vi "Meas Loop.vi"(8 "error in":errorcluster, 11 "meas in":T1={"swp cfg"={"N"=0, "R"=0, "f list"=[], "smpl delay"=0.0, "set delay"=0.0, "set delay np"=0.0, "meas root"=path "", "meas name"="", "meas a-index"=FALSE, "rnd sweep"=FALSE, "mode"=enum."Frequency", "swp mode"=enum."Linear", "avg"=0, "subrec"=0}, "bridge"={"type"=enum."TWM client", "TWM"={"pipe name"="", "parameters"=[], "handle"=0, "fixed aper [s]"=0.0, "f-list [Hz]"=[], "discrete f-list"=FALSE, "unc mode"=enum."None", "unc mcc"=0, "unc first"=FALSE}, "last f"=0.0, "bias comp"={"bias type"=enum."dummy", "VISA"="", "Enable"=FALSE, "channel qu"=[], "channel Uinit"=[]}}, "src"={"type"=enum."Tektronix AFG3101C", "afg"={"VISA"="", "const"=0.0, "gen DC"=FALSE, "ext ref"=FALSE}, "cDAQ dds"={"device"="", "channels"=[], "mclk source"="", "mclk [Hz]"=0.0, "use ext mclk"=FALSE, "fs [Hz]"=0.0, "block [s]"=0.0, "buf [s]"=0.0, "task"="", "cmd queue"=refnum, "proc ref"=refnum, "smpl clock out"="/cDAQ3/PFI0", "export smpl clock"=FALSE, "DC ofs [V]"=[]}, "gain [V/A]"=1.0, "F5xxx session"={"VISA"="", "mode"=enum."AC voltage", "Earth on"=FALSE, "Ext ref lock"=FALSE}}, "results"=refnum} {"src"."cDAQ dds"."channels" min=0 step=1; "bridge"."TWM"."f-list [Hz]" format="%#_6p"; "swp cfg"."f list"."bias" format="%#_3p"; "swp cfg"."f list"."level" format="%#_3p"; "swp cfg"."f list"."fs [Hz]" format="%#_5p"; "swp cfg"."f list"."time [s]" format="%#_3p"; "swp cfg"."f list"."f/fs" format="%#_3p"; "swp cfg"."f list"."periods" format="%#_3f"; "swp cfg"."f list"."f [Hz]" format="%#_5p"}) -> (0 "error out":errorcluster, 3 "meas out":T1={"swp cfg"={"N"=0, "R"=0, "f list"=[], "smpl delay"=0.0, "set delay"=0.0, "set delay np"=0.0, "meas root"=path "", "meas name"="", "meas a-index"=FALSE, "rnd sweep"=FALSE, "mode"=enum."Frequency", "swp mode"=enum."Linear", "avg"=0, "subrec"=0}, "bridge"={"type"=enum."TWM client", "TWM"={"pipe name"="", "parameters"=[], "handle"=0, "fixed aper [s]"=0.0, "f-list [Hz]"=[], "discrete f-list"=FALSE, "unc mode"=enum."None", "unc mcc"=0, "unc first"=FALSE}, "last f"=0.0, "bias comp"={"bias type"=enum."dummy", "VISA"="", "Enable"=FALSE, "channel qu"=[], "channel Uinit"=[]}}, "src"={"type"=enum."Tektronix AFG3101C", "afg"={"VISA"="", "const"=0.0, "gen DC"=FALSE, "ext ref"=FALSE}, "cDAQ dds"={"device"="", "channels"=[], "mclk source"="", "mclk [Hz]"=0.0, "use ext mclk"=FALSE, "fs [Hz]"=0.0, "block [s]"=0.0, "buf [s]"=0.0, "task"="", "cmd queue"=refnum, "proc ref"=refnum, "smpl clock out"="/cDAQ3/PFI0", "export smpl clock"=FALSE, "DC ofs [V]"=[]}, "gain [V/A]"=1.0, "F5xxx session"={"VISA"="", "mode"=enum."AC voltage", "Earth on"=FALSE, "Ext ref lock"=FALSE}}, "results"=refnum} {"src"."cDAQ dds"."channels" min=0 step=1; "bridge"."TWM"."f-list [Hz]" format="%#_6p"; "swp cfg"."f list"."bias" format="%#_3p"; "swp cfg"."f list"."level" format="%#_3p"; "swp cfg"."f list"."fs [Hz]" format="%#_5p"; "swp cfg"."f list"."time [s]" format="%#_3p"; "swp cfg"."f list"."f/fs" format="%#_3p"; "swp cfg"."f list"."periods" format="%#_3f"; "swp cfg"."f list"."f [Hz]" format="%#_5p"})   [LabVIEW 2013]
doc: "Main measurement loop."
uses:
  meas session.ctl
  Meas Sweep Config.ctl
  Meas Freq Info.ctl
  meas_swp_mode.ctl
  meas_sweep_flist_mode.ctl
  bridge/Bridge Session.ctl
  bridge/Bridge Type.ctl
  drivers/TWM client/TWM Session.ctl
  drivers/TWM client/TWM parameters.ctl
  drivers/TWM client/Meas Proc QWTB Uncertainty Mode.ctl
  bridge/Bridge Bias Session.ctl
  bridge/Bridge Bias Type.ctl
  source/Source Session.ctl
  source/Source Type.ctl
  drivers/AFG3101C/AFG3101C Session.ctl
  drivers/cDAQ DDS/cDAQ DDS Session.ctl
  drivers/cDAQ DDS/cDAQ DDS Setup.ctl
  drivers/Fluke 5XXX/top_lev/F5xxx_session.ctl
  drivers/Fluke 5XXX/top_lev/F5xxx_output_mode.ctl
  Meas Results.ctl
  bridge/Bridge Frequency Readings Data.ctl
  drivers/TWM client/Meas Proc QWTB Spectrum Data.ctl
  bridge/Bridge Sampling Setup.ctl
  varilib/varilib.lvlib
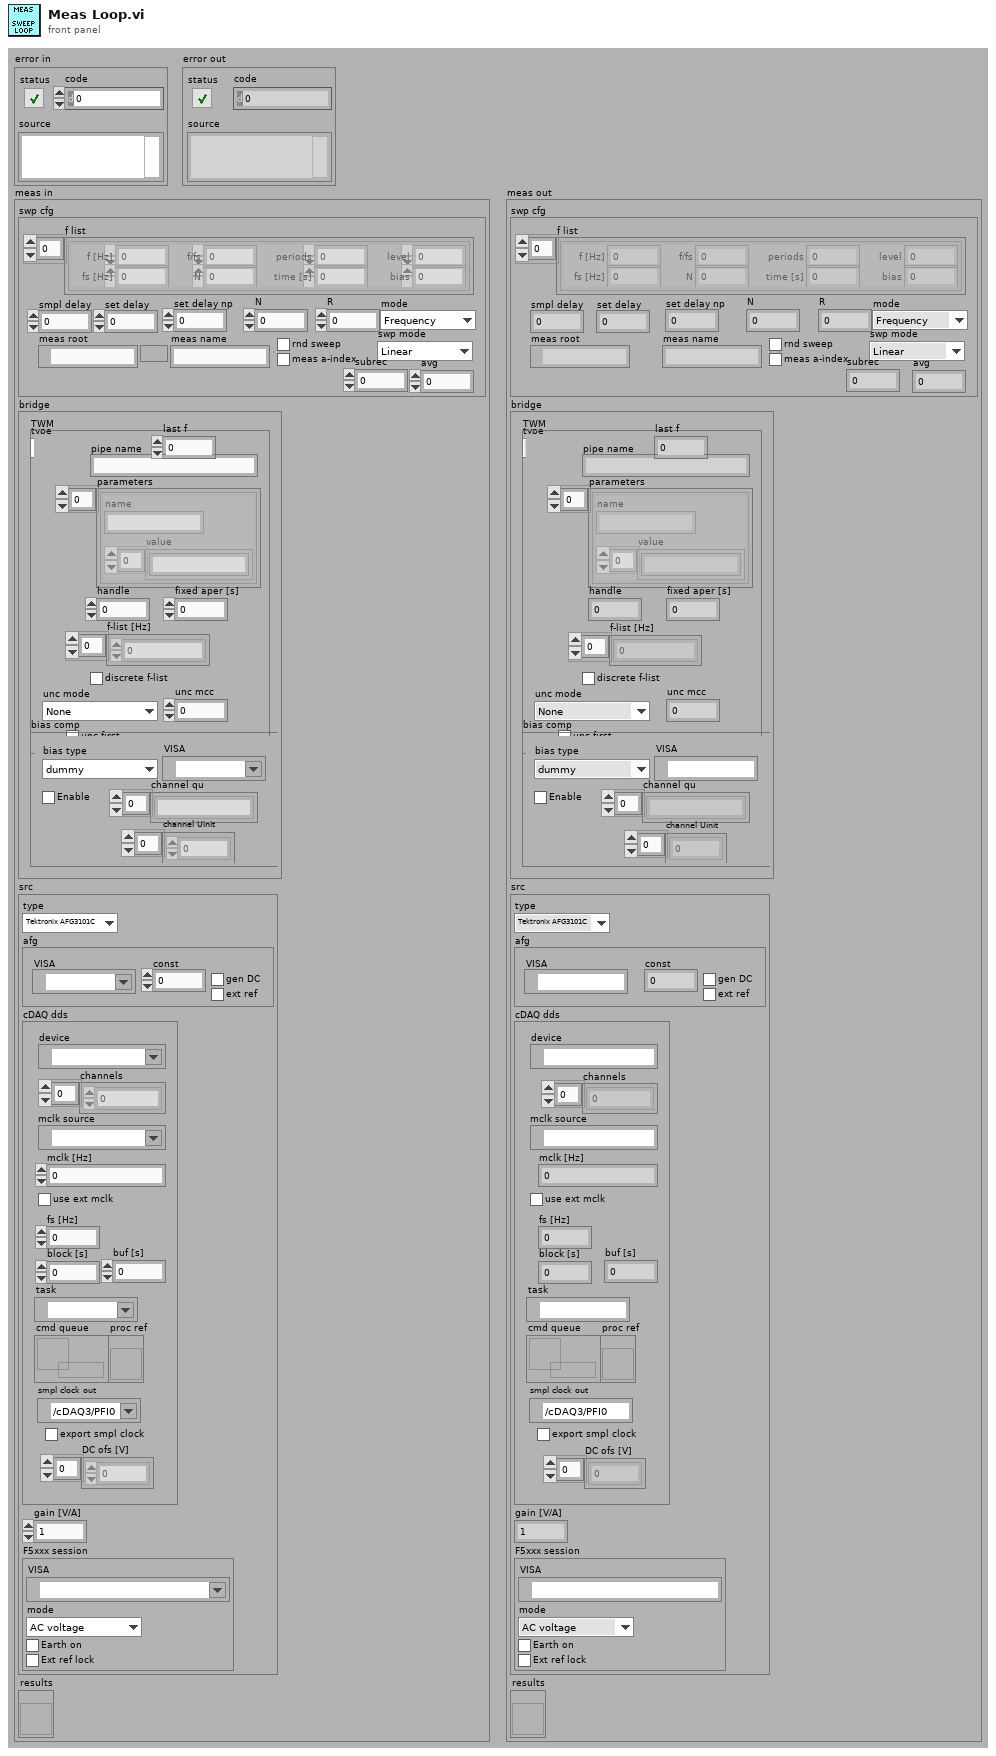
[diagram p1: front panel]
types:
  T1 = typedef "meas session.ctl" = cluster{"swp cfg":T2, "bridge":T6, "src":T13, "results":refnum<vi>}
  T2 = typedef "Meas Sweep Config.ctl" = cluster{"N":i32, "R":i32, "f list":T3[], "smpl delay":dbl, "set delay":dbl, "set delay np":dbl, "meas root":path, "meas name":string, "meas a-index":bool, "rnd sweep":bool, "mode":T4, "swp mode":T5, "avg":i32, "subrec":i32}
  T3 = typedef "Meas Freq Info.ctl" = cluster{"f [Hz]":dbl, "periods":dbl, "f/fs":dbl, "time [s]":dbl, "fs [Hz]":dbl, "N":i32, "level":dbl, "bias":dbl}
  T4 = typedef "meas_swp_mode.ctl" = enum16{"Frequency", "Level", "Bias"}
  T5 = typedef "meas_sweep_flist_mode.ctl" = enum16{"Linear", "Log10"}
  T6 = typedef "Bridge Session.ctl" = cluster{"type":T7, "TWM":T8, "last f":dbl, "bias comp":T11}
  T7 = typedef "Bridge Type.ctl" = enum16{"TWM client", "dummy"}
  T8 = typedef "TWM Session.ctl" = cluster{"pipe name":string, "parameters":T9[], "handle":i32, "fixed aper [s]":dbl, "f-list [Hz]":dbl[], "discrete f-list":bool, "unc mode":T10, "unc mcc":i32, "unc first":bool}
  T9 = typedef "TWM parameters.ctl" = cluster{"name":string, "value":string[]}
  T10 = typedef "Meas Proc QWTB Uncertainty Mode.ctl" = enum16{"None", "GUF", "Monte Carlo"}
  T11 = typedef "Bridge Bias Session.ctl" = cluster{"bias type":T12, "VISA":refnum<visa-resource-name>, "Enable":bool, "channel qu":string[], "channel Uinit":dbl[]}
  T12 = typedef "Bridge Bias Type.ctl" = enum16{"dummy", "CMI LiBbias V1.0"}
  T13 = typedef "Source Session.ctl" = cluster{"type":T14, "afg":T15, "cDAQ dds":T16, "gain [V/A]":dbl, "F5xxx session":T17}
  T14 = typedef "Source Type.ctl" = enum16{"Tektronix AFG3101C", "cDAQ DAC", "Fluke 5xxx", "Agilent 33120A", "dummy"}
  T15 = typedef "AFG3101C Session.ctl" = cluster{"VISA":refnum<visa-resource-name>, "const":dbl, "gen DC":bool, "ext ref":bool}
  T16 = typedef "cDAQ DDS Session.ctl" = cluster{"device":tag, "channels":i32[], "mclk source":tag, "mclk [Hz]":dbl, "use ext mclk":bool, "fs [Hz]":dbl, "block [s]":dbl, "buf [s]":dbl, "task":refnum<k21>, "cmd queue":refnum<queue>, "proc ref":refnum<vi>, "smpl clock out":tag, "export smpl clock":bool, "DC ofs [V]":dbl[]}
  T17 = typedef "F5xxx_session.ctl" = cluster{"VISA":refnum<visa-resource-name>, "mode":T18, "Earth on":bool, "Ext ref lock":bool}
  T18 = typedef "F5xxx_output_mode.ctl" = enum16{"AC voltage", "AC current"}
  T19 = typedef "Bridge Frequency Readings Data.ctl" = cluster{"Udut":dbl[], "Iref":dbl[], "Udc":dbl[], "Idc":dbl[], "mjr":dbl[], "mnr":dbl[], "mjr_sh":dbl[], "mnr_sh":dbl[], "u(mjr)":dbl[], "u(mnr)":dbl[], "ua2(mjr)":dbl[], "ua2(mnr)":dbl[], "n":i32, "f [Hz]":dbl}
  T20 = typedef "Meas Sequence Item.ctl" = cluster{"fid":i32, "n":i32, "newf":bool, "done":bool, "delay":dbl, "status":string, "path":path, "firstf":bool, "set bias":bool}
  T21 = typedef "Meas Results.ctl" = cluster{"freqs":T19[][], "locked":bool, "last fid":i32, "modified":bool, "mjr name":string, "mnr name":string, "last spectra":T22[][]}
  T22 = typedef "Meas Proc QWTB Spectrum Data.ctl" = cluster{"x":sgl[], "y":sgl[], "label":string}
  T23 = typedef "Bridge Sampling Setup.ctl" = cluster{"fs [Hz]":dbl, "samples":i32, "path":path, "f [Hz]":dbl, "avg":i32}
  T24 = typedef "Bridge Reading Data.ctl" = cluster{"Udut":dbl, "Iref":dbl, "Udc":dbl, "Idc":dbl, "mjr":dbl, "mnr":dbl, "mjr_sh":dbl, "mnr_sh":dbl, "u(mjr)":dbl, "u(mnr)":dbl, "ua(mjr)":dbl, "ua(mnr)":dbl, "mjr name":string, "mnr name":string, "session root":path, "spectra":T22[], "Udc_lo":dbl, "Udc_hi":dbl, "Udc_ref":dbl}
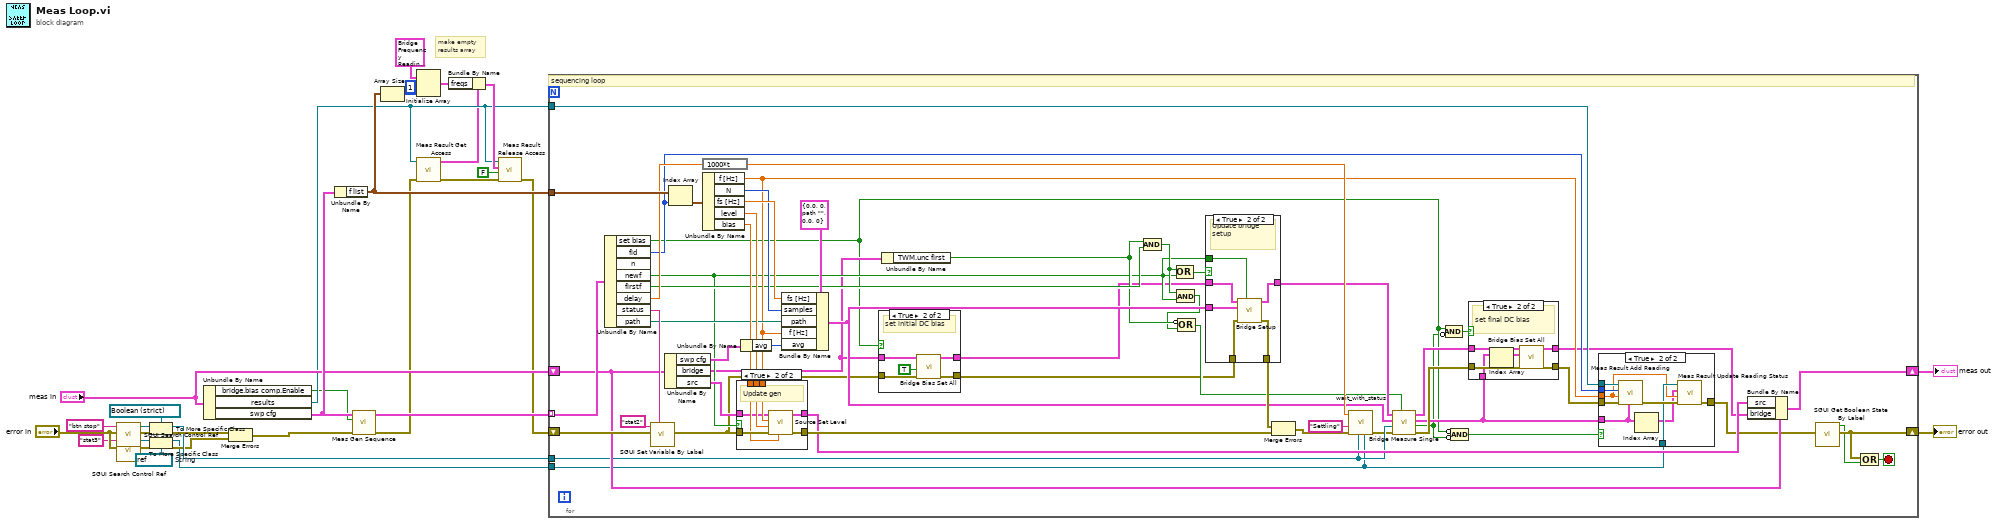
[diagram p0: block diagram]
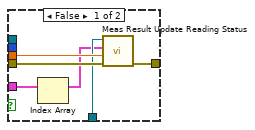
[diagram p4: hidden frame]
diagram:
  w15 = refnum<vi> refnum  # String
  # "make empty\nresults array"
  n1 = call "SGUI Search Control Ref.vi"("error in"="error in", "control label (empty)"="btn stop") -> ("error out"=w27:errorcluster, "control ref out"=w21:refnum<vi>)  [unwired: 7 in, 1 out]
  n2 = call "SGUI Search Control Ref.vi"("error in"="error in", "control label (empty)"="stat3") -> ("error out"=w26:errorcluster, "control ref out"=w17:refnum<vi>)  [unwired: 7 in, 1 out]
  n3 = To More Specific Class(target class=refnum<vi> refnum ("OK Button"), reference=w21, error in=w27) -> (specific class reference=w20:refnum<vi>, error out=w22:errorcluster)
  n4 = To More Specific Class(target class=w15, reference=w17, error in=w26) -> (specific class reference=w16:refnum<vi>, error out=w18:errorcluster)
  n5 = Unbundle By Name("meas in") -> ("bridge.bias comp.Enable"=w3:bool, "results"=w5:refnum<vi>, "swp cfg"=w30:T2)
  n6 = Merge Errors(w22, w18) -> (w25:errorcluster)
  n7 = Unbundle By Name(w30) -> ("f list"=w14:T3[])
  n8 = call "Meas Gen Sequence.vi"("error in"=w25, "DC bias compensate (False)"=w3, "sweep setup"=w30) -> ("error out"=w11:errorcluster, "sequence"=w32:T20[])  [unwired: 7 in]
  n9 = Array Size(array=w14) -> (size(s)=w13:i32)
  n10 = Initialize Array(T19 {"Udut"=[], "Iref"=[], "Udc"=[], "Idc"=[], "mjr"=[], "mnr"=[], "mjr_sh"=[], "mnr_sh"=[], "u(mjr)"=[], "u(mnr)"=[], "ua2(mjr)"=[], "ua2(mnr)"=[], "n"=0, "f [Hz]"=0.0} ("data"), 1 ("dimension size"), w13) -> (w8:T19[][])
  n11 = call "Meas Result Get Access.vi"("error in"=w11, "results ref"=w5) -> ("error out"=w12:errorcluster, "results data"=w1:T21)  [unwired: 8 in]
  n12 = Bundle By Name(cluster=w1, "freqs"=w8) -> (w7:T21)
  n13 = call "Meas Result Release Access.vi"("error in"=w12, "Release only (True)"=FALSE, "results data in"=w7, "results ref"=w5) -> ("error out"=w10:errorcluster)  [unwired: 7 in]
  n14 = for {
    shift-right: [w78] -> w31
    shift-left: w10 -> [w73]
    tunnel: w32 -> [w87] mode=indexing
    tunnel: w14 -> [w88]
    shift-right: [w62] -> w4
    shift-left: "meas in" -> [w64]
    tunnel: w20 -> [w55]
    tunnel: w16 -> [w54]
    tunnel: w5 -> [w61]
    stop <- w79 stop-if-true
    # "sequencing loop"
    n15 = Unbundle By Name(w87) -> ("set bias"=w35:bool, "fid"=w60:i32, "newf"=w47:bool, "firstf"=w52:bool, "delay"=w76:dbl, "status"=w72:string, "path"=w66:path)  [unwired: 1 out]
    n16 = call "SGUI Set Variable By Label.vi"("value (none)"=w72, "error in"=w73, "control label (none)"="stat2") -> ("error out"=w45:errorcluster)  [unwired: 7 in, 1 out]
    n17 = Unbundle By Name(w64) -> ("swp cfg"=w57:T2, "bridge"=w43:T6, "src"=w83:T13)
    n18 = Index Array(array=w88, index=w60) -> (element=w86:T3)
    n19 = expression code="1000*t"(w76) -> (w75:dbl)
    n20 = Unbundle By Name(w86) -> ("f [Hz]"=w59:dbl, "N"=w67:i32, "fs [Hz]"=w68:dbl, "level"=w85:dbl, "bias"=w84:dbl)
    n21 = case shown="True" w47 {
      tunnel: w45 -> [w127 w135]
      tunnel: w59 -> [_ w134]
      tunnel: w85 -> [_ w133]
      tunnel: w84 -> [_ w132]
      tunnel: w83 -> [w128 w131]
      tunnel: [w127 w130] -> w82
      tunnel: [w128 w129] -> w63
      frame False {
      }
      frame True {
        # "Update gen"
        n22 = call "Source Set Level.vi"("DC current [A]"=w132, "error in"=w135, "current [A]"=w133, "f [Hz]"=w134, "src in"=w131) -> ("error out"=w130:errorcluster, "src out"=w129:T13)  [unwired: 5 in]
      }
    }
    n23 = Unbundle By Name(w57) -> ("avg"=w56:i32)
    n24 = Bundle By Name(cluster=T23 {"fs [Hz]"=0.0, "samples"=0, "path"=path "", "f [Hz]"=0.0, "avg"=0} ("sampling"), "fs [Hz]"=w68, "samples"=w67, "path"=w66, "f [Hz]"=w59, "avg"=w56) -> (w65:T23)
    n25 = case shown="True" w35 {
      tunnel: w45 -> [w98 w103]
      tunnel: [w98 w102] -> w44
      tunnel: w43 -> [w97 w101]
      tunnel: [w97 w100] -> w42
      frame False {
      }
      frame True {
        # "set initial DC bias"
        n26 = call "Bridge Bias Set All.vi"("error in"=w103, "Set initial biases? (False)"=TRUE ("Set initial biases? (True)"), "bridge in"=w101) -> ("error out"=w102:errorcluster, "bridge out"=w100:T6)  [unwired: 7 in]
      }
    }
    n27 = Unbundle By Name(w43) -> ("TWM.unc first"=w51:bool)
    n28 = Compound Arithmetic op=AND(w51, w52) -> (w48:bool)
    n29 = Compound Arithmetic op=OR(w48, w47) -> (w49:bool)
    n30 = Compound Arithmetic op=AND(w48, w47) -> (w46:bool)
    n31 = Compound Arithmetic op=OR(invert w51, w46) -> (w50:bool)
    n32 = case shown="True" w49 {
      tunnel: w42 -> [w119 w126]
      tunnel: w44 -> [w120 w125]
      tunnel: [w120 w124] -> w81
      tunnel: [w119 w123] -> w70
      tunnel: w65 -> [_ w122]
      tunnel: w47 -> [_ w121]
      frame False {
      }
      frame True {
        # "Update bridge setup"
        n33 = call "Bridge Setup.vi"("allow uncertainty calculation (true)"=w121, "error in"=w125, "sampling"=w122, "bridge in"=w126) -> ("error out"=w124:errorcluster, "bridge out"=w123:T6)  [unwired: 6 in]
      }
    }
    n34 = Merge Errors(w81, w82) -> (w80:errorcluster)
    n35 = call "wait_with_status.vi"("stat ref"=w54, "stop ref"=w55, "error in"=w80, "comment"="Settling", "ms to wait"=w75) -> ("error out"=w53:errorcluster)  [unwired: 6 in]
    n36 = call "Bridge Measure Single.vi"("allow uncertainty calculation (true)"=w50, "error in"=w53, "stop ref (none)"=w55, "sampling"=w65, "bridge in"=w70) -> ("error out"=w40:errorcluster, "stoped?"=w33:bool, "reading per phase"=w37:T24[], "bridge out"=w39:T6)  [unwired: 3 in]
    n37 = Compound Arithmetic op=AND(w35, invert w33) -> (w36:bool)
    n38 = Compound Arithmetic op=AND(invert w35, invert w33) -> (w34:bool)
    n39 = case shown="True" w36 {
      tunnel: w40 -> [w90 w96]
      tunnel: [w90 w95] -> w41
      tunnel: w39 -> [w89 w94]
      tunnel: [w89 w93] -> w38
      tunnel: w37 -> [_ w92]
      frame False {
      }
      frame True {
        # "set final DC bias"
        n40 = Index Array(array=w92) -> (element=w91:T24)  [unwired: 1 in]
        n41 = call "Bridge Bias Set All.vi"("error in"=w96, "reading"=w91, "bridge in"=w94) -> ("error out"=w95:errorcluster, "bridge out"=w93:T6)  [unwired: 7 in]
      }
    }
    n42 = case shown="True" w34 {
      tunnel: w41 -> [w109 w118]
      tunnel: w61 -> [_ w117]
      tunnel: w60 -> [_ w116]
      tunnel: [w108 w114] -> w58
      tunnel: w54 -> [w105 w113]
      tunnel: w59 -> [w107 w111]
      tunnel: w37 -> [w106 w112]
      frame False {
        n43 = Index Array(array=w106) -> (element=w104:T24)  [unwired: 1 in]
        n44 = call "Meas Result Update Reading Status.vi"("error in"=w109, "f [Hz]"=w107, "reading"=w104, "str ref"=w105) -> ("error out"=w108:errorcluster)  [unwired: 7 in]
      }
      frame True {
        n45 = call "Meas Result Add Reading.vi"("reading per phase"=w112, "error in"=w118, "f [Hz]"=w111, "freq. id (default: 0)"=w116, "results ref"=w117) -> ("error out"=w115:errorcluster)  [unwired: 5 in, 1 out]
        n46 = Index Array(array=w112) -> (element=w110:T24)  [unwired: 1 in]
        n47 = call "Meas Result Update Reading Status.vi"("error in"=w115, "f [Hz]"=w111, "reading"=w110, "str ref"=w113) -> ("error out"=w114:errorcluster)  [unwired: 7 in]
      }
    }
    n48 = Bundle By Name(cluster=w64, "src"=w63, "bridge"=w38) -> (w62:T1)
    n49 = call "SGUI Get Boolean State By Label.vi"("error in"=w58) -> ("error out"=w78:errorcluster, "binary state out"=w77:bool)  [unwired: 8 in, 1 out]
    n50 = Compound Arithmetic op=OR(w78, w77) -> (w79:bool)
  }
  "error out" <- w31
  "meas out" <- w4
